vi "JYGetMirrorPos.vi"(3 "error in (no error)":errorcluster, 4 "Mirror":u16(ring) items=["Entrance", "Exit"], 5 "UniqueID":string, 6 "Refnum In":refnum<k7>) -> (0 "error out":errorcluster, 1 "Current Mirror Position":i32(ring) items=["EntranceMirror", "ExitMirror", "Front", "Side"], 2 "Refnum Out":refnum<k7>)   [LabVIEW 2009]
doc: "Get Mirror Pos.vi\n\nReturns the current position of the mirror.\n\n==============================\nInputs \n\nRefnumIn - LabView automation refnum for the mono\nUniqueID\nMirror Number \n\nError Cluster \n\n=========================\nOutputs -\n\nRefnum out - the automation refnum is passed through the VI\n\nMirror Position \n\nError Cluster"
panel:
  in  "Mode Select":bool
  out "UseUniqueId":bool
  # "Local / Front Panel Mode"
  # "Remote / Program Mode"
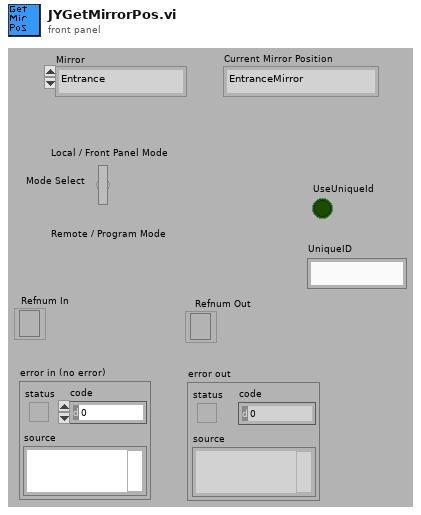
[diagram p1: front panel]
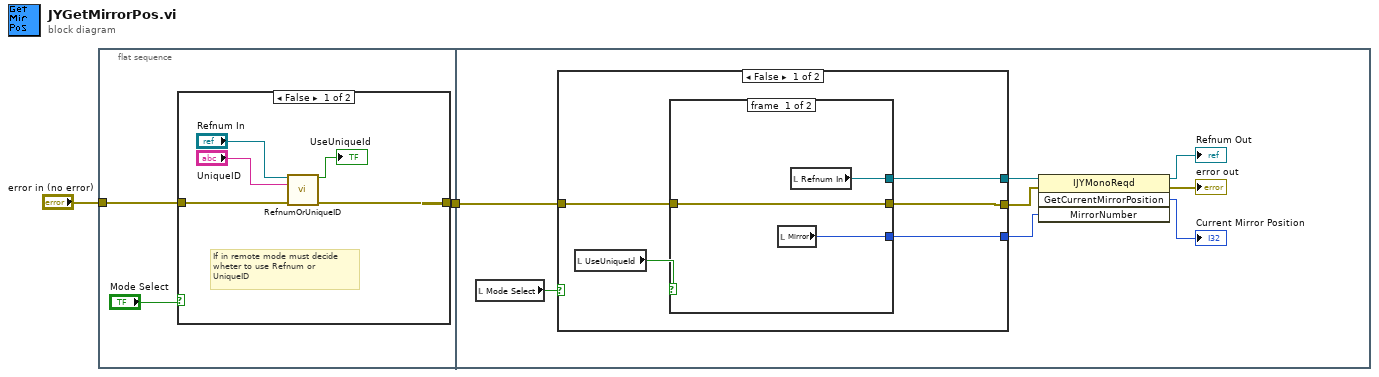
[diagram p0: block diagram]
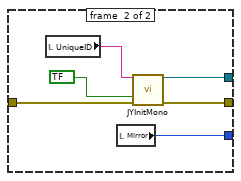
[diagram p3: hidden frame]
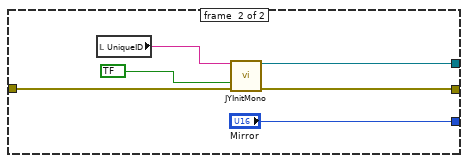
[diagram p4: hidden frame]
diagram:
  n1 = flat-sequence {
    tunnel: "error in (no error)" -> [w4]
    tunnel: [w3] -> w1
    tunnel: w1 -> [w18]
    frame #0 {
      n2 = case shown="False" "Mode Select" {
        tunnel: w4 -> [w8 w11]
        tunnel: [w6 w11] -> w3
        frame #0 {
          # "If in remote mode must decide\nwheter to use Refnum or \nUniqueID"
          n3 = call "RefnumOrUniqueID.vi"("Refnum IN"="Refnum In", "String in"="UniqueID", "error in (no error)"=w8) -> ("UseUniqueID"=→"UseUniqueId":bool, "error out"=w6:errorcluster)  [unwired: 11 out]
        }
        frame #1 {
        }
      }
    }
    frame #1 {
      n4 = local read "Mode Select"() -> (w19:bool)
      n5 = case shown="False" w19 {
        tunnel: w18 -> [w23 w39]
        tunnel: [w22 "Mirror"] -> w12
        tunnel: [w21 w35] -> w13
        tunnel: [w20 w34] -> w14
        frame #0 {
          n6 = local read "UseUniqueId"() -> (w24:bool)
          n7 = case shown="True" w24 {
            tunnel: w23 -> [w27 w33]
            tunnel: [w27 w30] -> w21
            tunnel: [w26 w29] -> w20
            tunnel: [w25 w28] -> w22
            frame #0 {
              n8 = local read "Mirror"() -> (w25:u16)
              n9 = local read "Refnum In"() -> (w26:refnum<k7>)
            }
            frame #1 {
              n10 = local read "UniqueID"() -> (w32:string)
              n11 = local read "Mirror"() -> (w28:u16)
              n12 = call "JYInitMono.vi"("Unique ID"=w32, "Force Init"=bool ?, "error in (no error)"=w33) -> ("Mono RefNum out"=w29:refnum<k7>, "error out"=w30:errorcluster)  [unwired: 1 in, 10 out]
            }
          }
        }
        frame #1 {
          n13 = local read "UniqueID"() -> (w38:string)
          n14 = call "JYInitMono.vi"("Unique ID"=w38, "Force Init"=bool ?, "error in (no error)"=w39) -> ("Mono RefNum out"=w34:refnum<k7>, "error out"=w35:errorcluster)  [unwired: 1 in, 10 out]
        }
      }
      n15 = invoke class="IJYMonoReqd" method="GetCurrentMirrorPosition"(reference=w14, error in=w13, "MirrorNumber"=w12) -> (reference out=→"Refnum Out":refnum<k7>, error out=→"error out":errorcluster, "GetCurrentMirrorPosition"=→"Current Mirror Position":i32)  [unwired: 1 in, 1 out]
    }
  }
